vi "Fetch Multiple Record Multiple Channel (Wfm).vi"(5 "FIFO Type":enum16{"FPGA to Host FIFO (U64)", "Generic"}(ring), 7 "Timeout (s)":i32=5, 8 "error in":errorcluster, 10 "Records to Fetch":i32, 11 "FPGA VI Reference In":refnum<k20>) -> (0 "error out":errorcluster, 2 "Acquired Data":waveform(dbl)[](array[waveform]), 3 "FPGA VI Reference Out":refnum<k20>, 4 "Elements Remaining":u32)   [LabVIEW 2011]
uses:
  <userlib>/FlexRIO Host Library/FlexRIO Host API/Acquire/Fetch/Fetch Acquired Data (U64).vi
  <vilib>/Utility/error.llb/Error Cluster From Error Code.vi
  <vilib>/rvi/errors/niLvFpgaAdjustHostInterfaceError.vi
  <vilib>/rvi/interface/nirviReadWriteControl/nirviReadWriteControl.xnode
  NiFpgaLv.dll
  <vilib>/rvi/interface/Simulation/niFpgaSimulationCallBeginRW.vi
  <userlib>/FlexRIO Host Library/FlexRIO Host Library (User).lvlib
panel:
  out "Data Acquired":i16[](array[numeric])
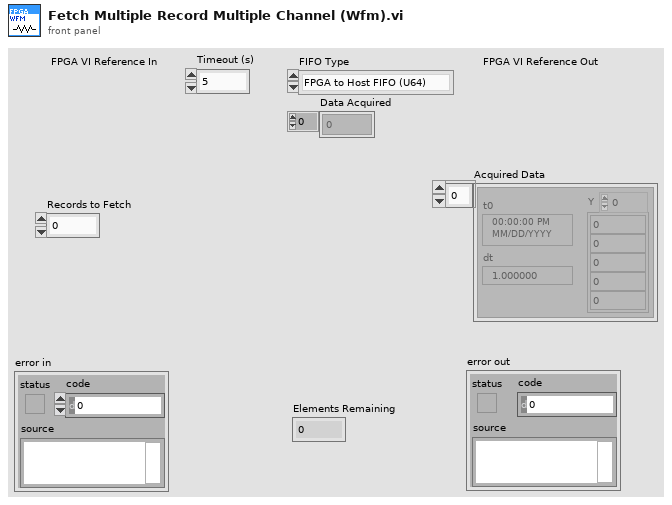
[diagram p1: front panel]
types:
  T1 = cluster{"Load Record Parameters?":bool, "Pre Trigger Samples":u16, "Samples per Record":u16, "Trigger Hold Off":u16, "Record Count":u16}
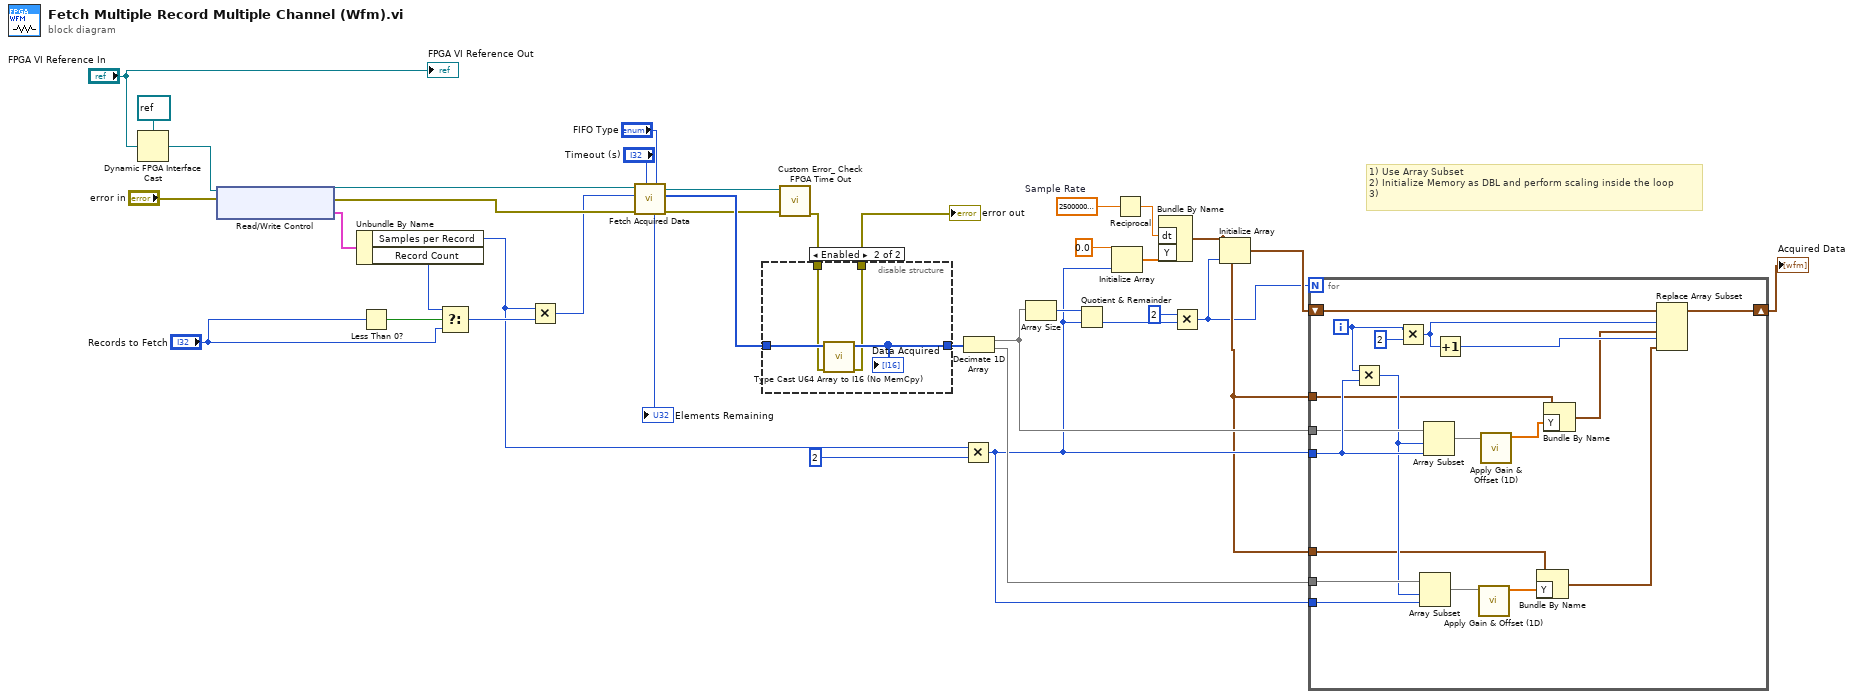
[diagram p0: block diagram]
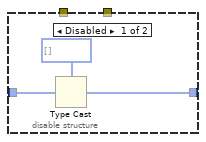
[diagram p2: hidden frame]
diagram:
  w4 = 250000000.0  # Sample Rate
  # "1) Use Array Subset\n2) Initialize Memory as DBL and perform scaling inside the loop\n3)"
  n1 = Dynamic FPGA Interface Cast(Session In=refnum<k20> refnum ("Type"), Type="FPGA VI Reference In") -> (Session Out=w34:refnum<k20>)
  n2 = xnode "Read/Write Control"("FPGA VI Reference In"=w34, "error in"="error in") -> ("FPGA VI Reference Out"=w29:refnum<k20>, "error out"=w28:errorcluster, "Record Parameters"=w33:T1)
  n3 = Unbundle By Name(w33) -> ("Samples per Record"=w20:u16, "Record Count"=w31:u16)
  n4 = Less Than 0?(x="Records to Fetch") -> (x < 0?=w32:bool)
  n5 = Select(t=w31, s=w32, f="Records to Fetch") -> (s? t:f=w21:i32)
  n6 = Multiply(x=w20, y=w21) -> (x*y=w27:i32)
  n7 = call-poly <userlib>:"Fetch Acquired Data.vi"("FIFO Type"="FIFO Type", "Timeout (s)"="Timeout (s)", "error out"=w28, "Samples"=w27, "FPGA Reference In"=w29) -> ("error out"=w15:errorcluster, "Data"=w24:u64[], "FPGA Reference Out"=w16:refnum<k20>, "Elements Remaining"=→"Elements Remaining":u32)  [unwired: 3 in]
  n8 = call <userlib>:"Custom Error_ Check FPGA Time Out.vi"("error in"=w15, "FPGA VI Reference In"=w16) -> ("error out"=w2:errorcluster)  [unwired: 8 in, 1 out]
  n9 = disable-structure shown="Enabled" {
    disable-tunnel: [w40 w43] -> w26
    disable-tunnel: w24 -> [w39 w44]
    disable-tunnel: w2 -> [_ w42]
    disable-tunnel: [_ w41] -> w1
    frame Disabled {
      n10 = Type Cast(type=i16[] [], x=w39) -> (*(type *) &x=w40:i16[])
    }
    frame Enabled {
      n11 = call <userlib>:"Type Cast U64 Array to I16 (No MemCpy).vi"("error in"=w42, "Input"=w44) -> ("error out"=w41:errorcluster, "Data Acquired"=w43:i16[])  [unwired: 8 in]
      "Data Acquired" <- w43
    }
  }
  "error out" <- w1
  n12 = Multiply(x=w20, y=u16 2) -> (x*y=w9:u16)
  n13 = Decimate 1D Array(w26) -> (w18:i16[], w11:i16[])
  n14 = Array Size(array=w18) -> (size(s)=w17:i32)
  n15 = Quotient & Remainder(x=w17, y=w9) -> (floor(x/y)=w13:i32)  [unwired: 1 out]
  n16 = Initialize Array(0.0 ("element"), w9) -> (w10:dbl[])
  n17 = Reciprocal(x=w4) -> (1/x=w3:dbl)
  n18 = Bundle By Name("dt"=w3, "Y"=w10) -> (w7:waveform(dbl))  [unwired: 1 in]
  n19 = Multiply(x=2, y=w13) -> (x*y=w5:i32)
  n20 = Initialize Array(w7, w5) -> (w8:waveform(dbl)[])
  n21 = for {
    N: w5 -> [_]
    tunnel: w18 -> [w62]
    tunnel: w9 -> [w63]
    tunnel: w11 -> [w61]
    tunnel: w9 -> [w59]
    shift-right: [w57] -> w6
    shift-left: w8 -> [w58]
    tunnel: w7 -> [w50]
    tunnel: w7 -> [w47]
    i -> [w54]
    n22 = Multiply(x=w54, y=w63) -> (x*y=w60:i32)
    n23 = Multiply(x=w54, y=2) -> (x*y=w52:i32)
    n24 = Array Subset(array=w61, index=w60, length=w59) -> (w55:i16[])
    n25 = Array Subset(array=w62, index=w60, length=w63) -> (w56:i16[])
    n26 = Increment(x=w52) -> (x+1=w51:i32)
    n27 = call <userlib>:"Apply Gain & Offset (1D).vi"("Raw Data"=w55) -> ("Scaled Data"=w48:dbl[])  [unwired: 10 in]
    n28 = call <userlib>:"Apply Gain & Offset (1D).vi"("Raw Data"=w56) -> ("Scaled Data"=w49:dbl[])  [unwired: 10 in]
    n29 = Bundle By Name(cluster=w47, "Y"=w48) -> (w45:waveform(dbl))
    n30 = Bundle By Name(cluster=w50, "Y"=w49) -> (w46:waveform(dbl))
    n31 = Replace Array Subset(array=w58, new element #1=w46, index #1=w52, new element #2=w45, index #2=w51) -> (w57:waveform(dbl)[])
  }
  "Acquired Data" <- w6
  "FPGA VI Reference Out" <- "FPGA VI Reference In"
